vi "WPI_GyroRomiReset.vi"(8 "error in (no error)":errorcluster, 11 "GyroDevRef":T1={"DevStatus"={"status"=FALSE, "code"=0, "source"=""}, "Analog Channel"=enum."AI 1", "Gain (VoltsPerDegree/Second)"=0.0, "Gyro Type"=enum."Analog", "Handle"=0, "SPI Bus"=enum."Invalid", "Device Found"=FALSE, "Sample Rate"=1.0, "Calibrate On Open"=FALSE, "Offset"=0.0} {"Sample Rate" min=0.25 max=100.0 step=0.25}) -> (0 "error out":errorcluster, 3 "GyroDevRef":T1={"DevStatus"={"status"=FALSE, "code"=0, "source"=""}, "Analog Channel"=enum."AI 1", "Gain (VoltsPerDegree/Second)"=0.0, "Gyro Type"=enum."Analog", "Handle"=0, "SPI Bus"=enum."Invalid", "Device Found"=FALSE, "Sample Rate"=1.0, "Calibrate On Open"=FALSE, "Offset"=0.0} {"Sample Rate" min=0.25 max=100.0 step=0.25})   [LabVIEW 2019]
doc: "Resets the gyroscope to a heading of zero. Use this VI to recalibrate the gyroscope after significant drift.\n\nThis software is licensed. Open the labview\\readme\\WPI Robotics Library Open Source License.txt file for more information."
uses:
  <vilib>/Rock Robotics/WPI/Simulation/Protocol/Devices/Gyro/Gyro Update Ops.ctl
  <vilib>/Rock Robotics/SystemInterfaces/AI/FPGA_AIChannel.ctl
  <vilib>/Rock Robotics/WPI/Gyro/WPI_GyroDevRef.ctl
  <vilib>/Rock Robotics/SystemInterfaces/spilib/spi_bus.ctl
panel:
  # "Analog"
  # "XRS"
  # "Analog"
  # "XRS"
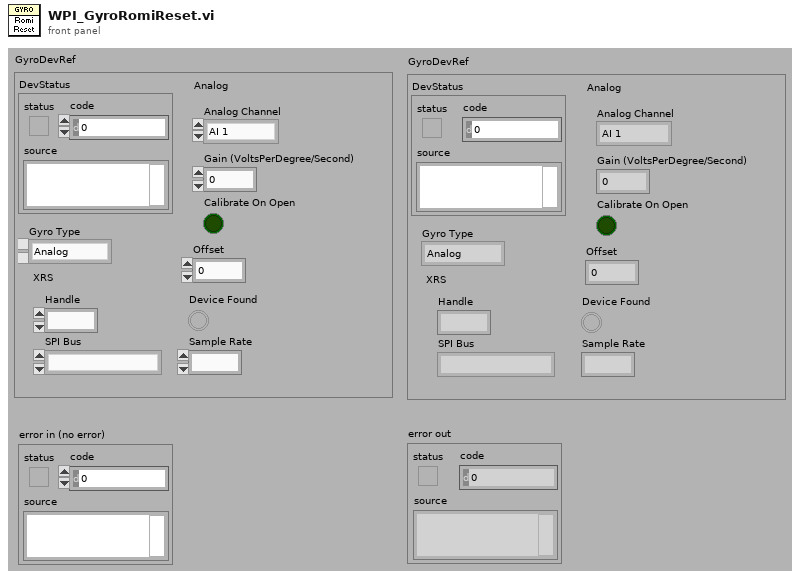
[diagram p1: front panel]
types:
  T1 = typedef "WPI_GyroDevRef.ctl" = cluster{"DevStatus":errorcluster, "Analog Channel":T2, "Gain (VoltsPerDegree/Second)":dbl, "Gyro Type":enum16{"Analog", "XRS450"}, "Handle":i32, "SPI Bus":T3, "Device Found":bool, "Sample Rate":dbl, "Calibrate On Open":bool, "Offset":dbl}
  T2 = typedef "FPGA_AIChannel.ctl" = enum8{"AI 0", "AI 1", "AI 2", "AI 3", "AI MXP 0", "AI MXP 1", "AI MXP 2", "AI MXP 3", "Invalid"}
  T3 = typedef "spi_bus.ctl" = enum16{"SPI On-Board, CS0", "SPI On-Board, CS1", "SPI On-Board, CS2", "SPI On-Board, CS3", "SPI MXP", "Invalid"}
  T4 = typedef "Gyro Update Ops.ctl" = enum16{"get", "delete", "JSON update", "set  name", "transmit initial", "reset", "set init", "set offsetX", "set offsetY", "set offsetZ", "set gain"}
  T5 = typedef "Gyro proto.ctl" = cluster{"type":string, "device":string, "name":string, "data":T6}
  T6 = typedef "Gyro Data proto.ctl" = cluster{"<init":bool, ">connected":bool, "<offsetX":dbl, "<offsetY":dbl, "<offsetZ":dbl, ">angleX":dbl, ">angleY":dbl, ">angleZ":dbl, ">rateX":dbl, ">rateY":dbl, ">rateZ":dbl, "<gain":dbl}
  T7 = cluster{">angleX":dbl, ">angleY":dbl, ">angleZ":dbl}
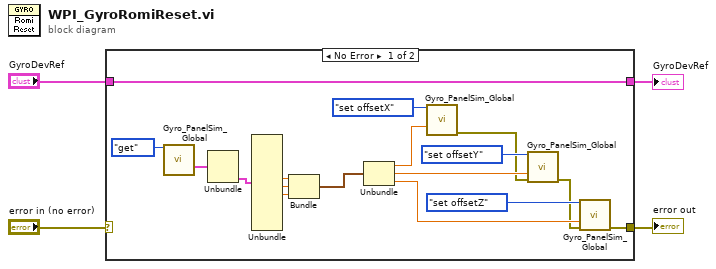
[diagram p0: block diagram]
diagram:
  n1 = case shown="No Error" "error in (no error)" {
    selector: "error in (no error)" -> [_ w23]
    tunnel: "GyroDevRef" -> [w21 w22]
    tunnel: [w21 w22] -> w3
    tunnel: [w17 w23] -> w1
    frame No Error {
      n2 = call <vilib>:"Gyro_PanelSim_Global.vi"("Menu"=Gyro_Update_Ops."get") -> ("Value out"=w15:T5)  [unwired: 13 in, 1 out]
      n3 = Unbundle(w15) -> ("data"=w14:T6)  [unwired: 3 out]
      n4 = Unbundle(w14) -> (">angleX"=w13:dbl, ">angleY"=w12:dbl, ">angleZ"=w11:dbl)  [unwired: 9 out]
      n5 = Bundle(">angleX"=w13, ">angleY"=w12, ">angleZ"=w11) -> (w5:T7)  [unwired: 1 in]
      n6 = Unbundle(w5) -> (">angleX"=w10:dbl, ">angleY"=w9:dbl, ">angleZ"=w8:dbl)
      n7 = call <vilib>:"Gyro_PanelSim_Global.vi"("Menu"=Gyro_Update_Ops."set offsetX", "Numeric Value"=w10) -> ("error out"=w6:errorcluster)  [unwired: 12 in, 1 out]
      n8 = call <vilib>:"Gyro_PanelSim_Global.vi"("Menu"=Gyro_Update_Ops."set offsetY", "Numeric Value"=w9, "error in (no error)"=w6) -> ("error out"=w7:errorcluster)  [unwired: 11 in, 1 out]
      n9 = call <vilib>:"Gyro_PanelSim_Global.vi"("Menu"=Gyro_Update_Ops."set offsetZ", "Numeric Value"=w8, "error in (no error)"=w7) -> ("error out"=w17:errorcluster)  [unwired: 11 in, 1 out]
    }
    frame Error {
    }
  }
  "GyroDevRef" <- w3
  "error out" <- w1
